vi "Data Access.vi"(8 "error in (no error)":errorcluster, 10 "Data Access Handler":refnum<class "Data Access Handler.lvclass">, 11 "Test Double Data Tracker in":refnum<class "Test Double Data Tracker.lvclass">) -> (0 "error out":errorcluster, 3 "Test Double Data Tracker out":refnum<class "Test Double Data Tracker.lvclass">)   [LabVIEW 2020, in "Test.lvlib" / "Test Double Data Tracker.lvclass"]
doc: "Expose class private data to the front panel while letting the Data Access Handler class act on the data."
uses:
  Test Double Data Tracker.lvclass
  PPL/HDH.Actor Framework.Core.Msg.lvlibp/Flex Msg/Data Access Handlers/Data Access Handler/Data Access Handler.lvclass
  PPL/HDH.Actor Framework.Core.Data Tracker.lvlibp/Messages for this Actor/Data Tracker Msg/Data Tracker Msg.lvclass
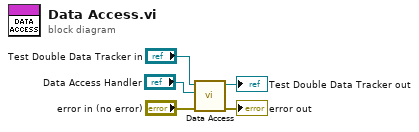
[diagram p0: block diagram]
diagram:
  n1 = call-parent "Data Access.vi"("error in (no error)"="error in (no error)", "Data Access Handler"="Data Access Handler", "Data Tracker Msg in"="Test Double Data Tracker in") -> ("error out"=→"error out":errorcluster, "Data Tracker Msg out"=→"Test Double Data Tracker out":refnum<class "Test Double Data Tracker.lvclass">)  [unwired: 7 in]
